vi "string array to spreadsheet string - no eol.vi"(1 "string array":string[](array[string])) -> (0 "spreadsheet string - no eol":string)   [LabVIEW 2017]
doc: "____________________________________________\nDIPC 692 Daemon API 10.0.0.1\nSam Tee - Dyson Technology Ltd\nCopyright (c) 2024, Dyson Technology Ltd"
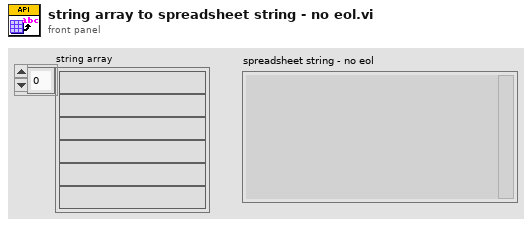
[diagram p1: front panel]
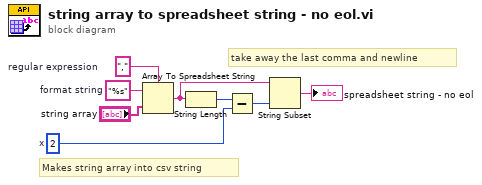
[diagram p0: block diagram]
diagram:
  w1 = ","  # regular expression
  w8 = 2  # x
  w3 = "%s"  # format string
  # "Makes string array into csv string"
  # "take away the last comma and newline"
  n1 = Array To Spreadsheet String(delimiter (Tab)=w1, array="string array", 3:w3) -> (spreadsheet string=w6:string)
  n2 = String Length(string=w6) -> (length=w4:i32)
  n3 = Subtract(x=w4, y=w8) -> (x-y=w5:i32)
  n4 = String Subset(string=w6, length (rest)=w5) -> (substring=→"spreadsheet string - no eol":string)  [unwired: 1 in]
